vi "Assert XML Serialize.vi"() -> ()   [LabVIEW 2015, in "XML Project.lvclass"]
uses:
  XML Project.lvclass
  <vilib>/xml/Close Reference(Node).vi
  <vilib>/xml/NI_XML.lvlib
  <resource>/objmgr/DOMUserDefRef.rc
panel:
  out "XML":string
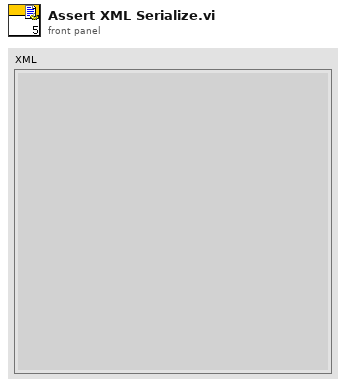
[diagram p1: front panel]
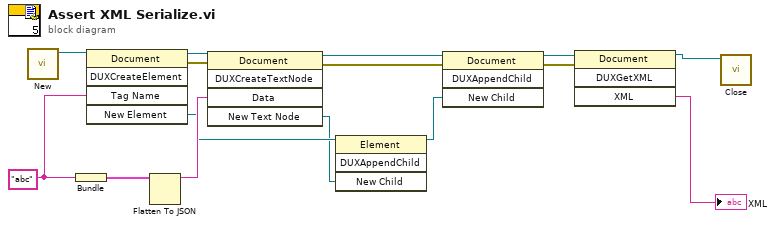
[diagram p0: block diagram]
diagram:
  w12 = "abc" ("Tag Name")
  n1 = call <vilib>:"New.vi"() -> ("DOM document out"=w15:refnum<k20>)  [unwired: 8 in, 1 out]
  n2 = Bundle("Tag Name"=w12) -> (w11:cluster{"Tag Name":string})  [unwired: 1 in]
  n3 = invoke class="Document" method="DUXCreateElement"(reference=w15, "Tag Name"=w12) -> (reference out=w14:refnum<k20>, error out=w13:errorcluster, "New Element"=w9:refnum<k20>)  [unwired: 3 in, 2 out]
  n4 = Flatten To JSON(anything=w11) -> (JSON string=w10:string)  [unwired: 2 in, 1 out]
  n5 = invoke class="Document" method="DUXCreateTextNode"(reference=w14, error in=w13, "Data"=w10) -> (reference out=w7:refnum<k20>, error out=w6:errorcluster, "New Text Node"=w8:refnum<k20>)  [unwired: 2 in, 2 out]
  n6 = invoke class="Element" method="DUXAppendChild"(reference=w9, "New Child"=w8) -> (reference out=w5:refnum<k20>)  [unwired: 2 in, 3 out]
  n7 = invoke class="Document" method="DUXAppendChild"(reference=w7, error in=w6, "New Child"=w5) -> (reference out=w4:refnum<k20>, error out=w3:errorcluster)  [unwired: 1 in, 2 out]
  n8 = invoke class="Document" method="DUXGetXML"(reference=w4, error in=w3) -> (reference out=w1:refnum<k20>, "XML"=→"XML":string)  [unwired: 2 in, 2 out]
  n9 = call-poly <vilib>:"Close.vi"("node"=w1) -> ()  [unwired: 8 in, 1 out]
